vi "Thermo.vi"(1 "Temp Scale":bool) -> (0 "Temperature":dbl(slide) scale=0.0..100.0 scale format="%.1f")   [LabVIEW 2020]
doc: "This VI is the solution to an exercise in the LabVIEW Basics I course.\n\nIt simulates measuring a temperature using the temperature sensor on the DAQ Signal Accessory.\n\nIf you have a DAQ board or a DAQ Signal Accessory, then use the Thermometer VI instead."
panel:
  # "deg C\n\ndeg F"
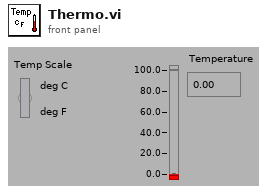
[diagram p1: front panel]
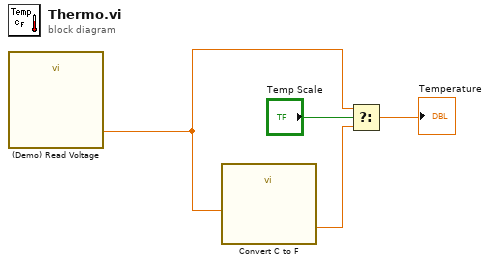
[diagram p0: block diagram]
diagram:
  n1 = call "(Demo) Read Voltage.vi"() -> ("voltage"=w1:dbl)  [unwired: 6 in, 1 out]
  n2 = call "Convert C to F.vi"("deg C"=w1) -> ("deg F"=w2:dbl)
  n3 = Select(t=w1, s="Temp Scale", f=w2) -> (s? t:f=→"Temperature":dbl)
